vi "VI.open_lua.vi"(5 "LuaVIEW reference":T1) -> (15 "error out":errorcluster)   [LabVIEW 2012]
doc: "Opens a VI object. This function uses the standard LabVIEW Open VI Refence node to obtain a VI reference that is subsequently packaged into a LuaVIEW object with attached methods. When a VI with the same name is already loaded in memory, a reference to that VI is returned. When the path is relative, the VI will be searched for relative to the directory containing the calling task's main script. If the VI is not found there or if the calling script is not a task, the plug-in will be searched for relative to the resource base path. When running as a built application, the application executable will also be searched.\n\nWhen the referenced VI is a template that is not already in memory, a clone of the template with its own front panel and data space will be instantiated. When \"prepare for reentrant run\" is requested for a non-template reentrant VI via the options bitset, the VI will be set up to be runnable with a new data space instance but not a front panel instance.\n\nBeware that when the top-level context (such as a task) from which the reference was opened is stopped, the VI reference is automatically closed by LabVIEW unless it was passed along via the \"auto dispose ref\" option of the run method .\nParameters:\nstr:path, path to the VI to open.\n[I32:options], options bitset as detailed in the LabVIEW Open VI Reference documentation. Defaults to zero when not specified.\nResults:\nobj:vi, a VI object.\nErrors:\nVI not found."
uses:
  typedefs/t_LuaVIEW Reference.ctl
  subvis/private/LuaVIEW Pull (path).vi
  subvis/private/LuaVIEW Pull (I32).vi
  subvis/private/LuaVIEW Push (object).vi
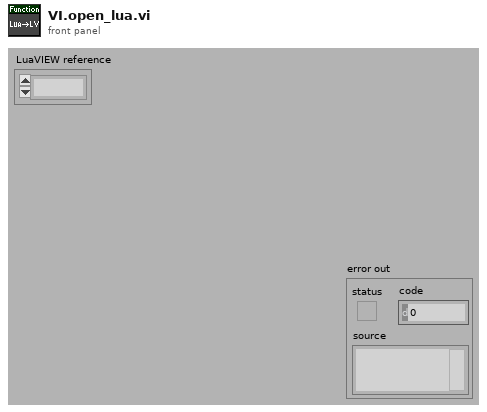
[diagram p1: front panel]
types:
  T1 = typedef "t_LuaVIEW Reference.ctl" = refnum<k1>
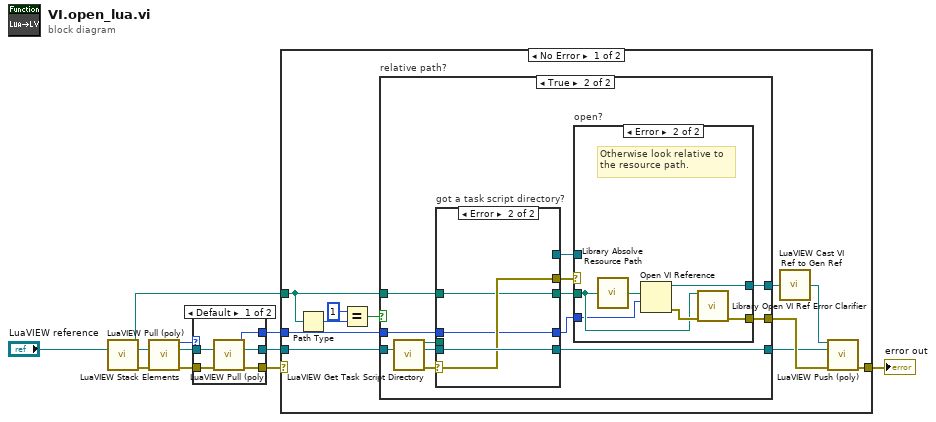
[diagram p0: block diagram]
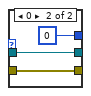
[diagram p2: hidden frame]
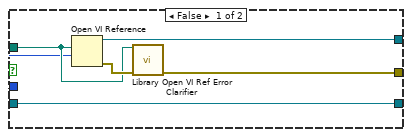
[diagram p3: hidden frame]
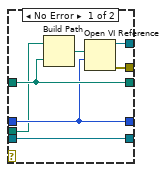
[diagram p5: hidden frame]
diagram:
  n1 = call-poly "LuaVIEW Pull (poly).vi"("LuaVIEW reference in"="LuaVIEW reference") -> ("path"=w10:path, "LuaVIEW reference out"=w5:T1, "error out"=w6:errorcluster)  [unwired: 12 in]
  n2 = call "LuaVIEW Stack Elements.vi"("LuaVIEW reference in"=w5, "error in (no error)"=w6) -> ("elements"=w9:i32, "LuaVIEW reference out"=w7:T1, "error out"=w8:errorcluster)  [unwired: 11 in]
  n3 = case shown="Default" w9 {
    tunnel: w8 -> [w16 w18]
    tunnel: w7 -> [w15 w19]
    tunnel: [w14 w19] -> w4
    tunnel: [w13 0] -> w2
    tunnel: [w12 w18] -> w3
    frame Default {
      n4 = call-poly "LuaVIEW Pull (poly).vi"("LuaVIEW reference in"=w15, "error in (no error)"=w16) -> ("I32"=w13:i32, "LuaVIEW reference out"=w14:T1, "error out"=w12:errorcluster)  [unwired: 11 in]
    }
    frame 0 {
    }
  }
  n5 = case shown="No Error" w3 {
    selector: w3 -> [_ w69]
    tunnel: [w22 w69] -> w1
    tunnel: w10 -> [w20 _]
    tunnel: w4 -> [w27 _]
    tunnel: w2 -> [w26 _]
    frame No Error {
      n6 = Path Type(1:w20) -> (0:w30:i16)
      n7 = Equal?(x=i16 1, y=w30) -> (x = y?=w28:bool)
      n8 = case "relative path?" shown="True" w28 {
        tunnel: w27 -> [w36 w49]
        tunnel: [w36 w45] -> w21
        tunnel: w20 -> [w34 w47]
        tunnel: [w33 w40] -> w23
        tunnel: [w32 w39] -> w24
        tunnel: w26 -> [w31 w38]
        frame False {
          n9 = Open VI Reference(vi path=w34, options=w31) -> (vi reference=w32:refnum<vi>, error out=w35:errorcluster)  [unwired: 4 in]
          n10 = call "Library Open VI Ref Error Clarifier.vi"("VI path"=w34, "called VI error (no error)"=w35) -> ("error out"=w33:errorcluster)  [unwired: 13 in]
        }
        frame True {
          n11 = call "LuaVIEW Get Task Script Directory.vi"("LuaVIEW reference in"=w49) -> ("task script directory"=w48:path, "LuaVIEW reference out"=w46:T1, "error out"=w44:errorcluster)  [unwired: 12 in]
          n12 = case "got a task script directory?" shown="Error" w44 {
            selector: w44 -> [_ w67]
            tunnel: w48 -> [w58 _]
            tunnel: w47 -> [w62 w66]
            tunnel: w46 -> [w63 w68]
            tunnel: [w63 w68] -> w45
            tunnel: [w62 w66] -> w41
            tunnel: [w61 w67] -> w43
            tunnel: [w60 _] -> w42
            tunnel: w38 -> [w59 w65]
            tunnel: [w59 w65] -> w37
            frame No Error {
              n13 = Build Path(base path=w58, name or relative path=w62) -> (appended path=w64:path)
              n14 = Open VI Reference(vi path=w64, options=w59) -> (vi reference=w60:refnum<vi>, error out=w61:errorcluster)  [unwired: 4 in]
            }
            frame Error {
            }
          }
          n15 = case "open?" shown="Error" w43 {
            selector: w43 -> [w50 _]
            tunnel: w42 -> [w51 _]
            tunnel: w41 -> [_ w54]
            tunnel: [w50 w55] -> w40
            tunnel: [w51 w53] -> w39
            tunnel: w37 -> [_ w52]
            frame No Error {
            }
            frame Error {
              # "Otherwise look relative to\nthe resource path."
              n16 = call "Library Absolve Resource Path.vi"("path in"=w54) -> ("absolved path"=w57:path)  [unwired: 14 in]
              n17 = Open VI Reference(vi path=w57, options=w52) -> (vi reference=w53:refnum<vi>, error out=w56:errorcluster)  [unwired: 4 in]
              n18 = call "Library Open VI Ref Error Clarifier.vi"("VI path"=w54, "called VI error (no error)"=w56) -> ("error out"=w55:errorcluster)  [unwired: 13 in]
            }
          }
        }
      }
      n19 = call "LuaVIEW Cast VI Ref to Gen Ref.vi"("refnum in"=w24) -> ("refnum out"=w25:refnum<vi>)  [unwired: 14 in]
      n20 = call-poly "LuaVIEW Push (poly).vi"("object refnum"=w25, "LuaVIEW reference in"=w21, "error in (no error)"=w23) -> ("error out"=w22:errorcluster)  [unwired: 11 in, 1 out]
    }
    frame Error {
    }
  }
  "error out" <- w1
